vi "getStatus.vi"(8 "error in (no error)":errorcluster, 11 "Instrument.Lockin":refnum<class "Instrument.Lockin.lvclass">) -> (0 "error out":errorcluster, 2 "state":T1=enum."created", 3 "Instrument.Lockin":refnum<class "Instrument.Lockin.lvclass">)   [LabVIEW 2019, in "Instrument.Lockin.lvclass"]
doc: "Get the lockin status {created, started, stopped, idle, sweeping}\n\nIf address=\"\", this API reads from localhost\nIf address is remote lockin, you need to add this computer to allowed whitelist on the lockin computer you are trying to access."
uses:
  Instrument.Lockin.lvclass
  <userlib>/LevyLab/Instrument Framework/Instrument Types/Lockin/Typedefs/LockinAPI.getState.states--enum.ctl
  <userlib>/LevyLab/Instrument Framework/Instrument Types/Lockin/Instrument.LockinAPI.lvclass
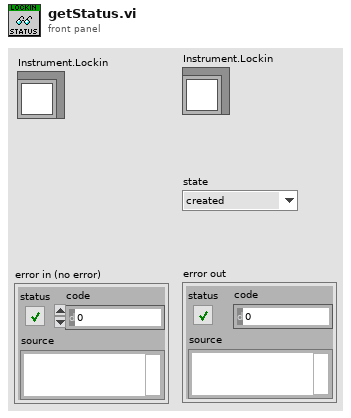
[diagram p1: front panel]
types:
  T1 = typedef "Instrument.LockinAPI.lvclass/LockinAPI.getState.states--enum.ctl" = enum16{"idle", "created", "started", "stopped", "sweeping"}
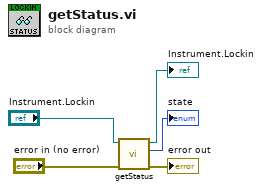
[diagram p0: block diagram]
diagram:
  n1 = call-parent "getStatus.vi"("error in (no error)"="error in (no error)", "Instrument.LockinAPI in"="Instrument.Lockin") -> ("error out"=→"error out":errorcluster, "state"=→"state":T1, "Instrument.LockinAPI out"=→"Instrument.Lockin":refnum<class "Instrument.Lockin.lvclass">)  [unwired: 7 in]
